vi "72 MP_Setting a servo.vi"() -> ()   [LabVIEW 2024]
uses:
  <userlib>/1. Examples/_Subs/OpenDiagram/Open_XControl.xctl
  <vilib>/Instr/_visa.llb/VISA Configure Serial Port (Instr).vi
panel:
  in  "OpenDiag":refnum<vi>(xcontrol)
  out "position read":u8=100
  in  "Position":u8(slide)=98 scale=0.0..180.0
  in  "MicroPython code":string="'''\nhttps://docs.micropython.org/en/latest/pyboard/tutorial/servo.html\n     \nconnections: \nGround (B) - GND \nPower  (R)   - 3V3 \nNC\nSignal -  pin X1\n'''\n\nimport pyb,utime,machine\n\nmachine.Pin('EN_3V3').on()\n\nusb = pyb.USB_VCP()\nservo1 = pyb.Servo(1)   # pix X1 \n\nwhile True:\n     utime.sleep_ms(10)\n     if usb.any():\n          reply = ord(usb.read())\n          #set the angle\n          servo1.angle(reply)\n          usb.send('%d \\n'%(reply))"
  in  "stop":bool
  out "Connected":bool
  in  "MicroPython Port":refnum<visa-resource-name>="ASRL96::INSTR"
  # "02 MicroPython Setting a Servo\nThis code takes will send a desired angle out to the device\n\nInstructions:\n1. Download the MicroPython Code into your device by saving it as main.py on your device\n2. restart your device\n3. Select the device port \n4. Hit Run - and watch the servo change position when you move the slider"
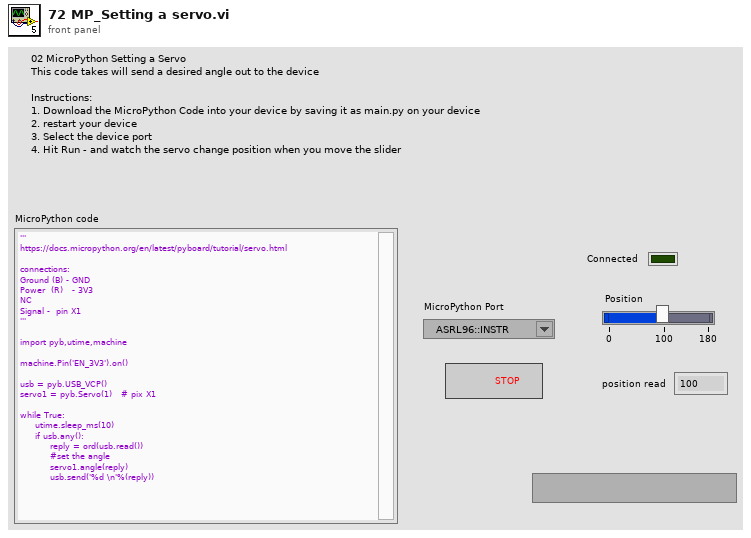
[diagram p1: front panel]
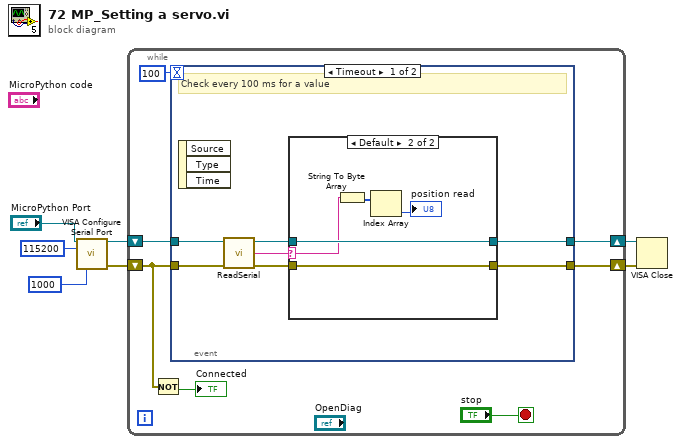
[diagram p0: block diagram]
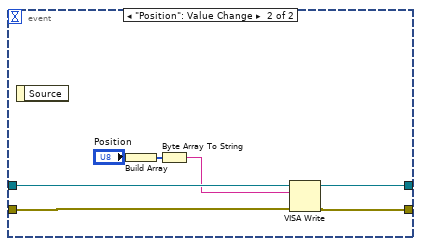
[diagram p3: hidden frame]
diagram:
  n1 = call-poly "VISA Configure Serial Port"("VISA resource name"="MicroPython Port", "timeout (10sec)"=u32 1000, "baud rate (9600)"=u32 115200) -> ("VISA resource name out"=w6:refnum<visa-resource-name>, "error out"=w5:errorcluster)  [unwired: 11 in]
  n2 = while {
    shift-right: [w12] -> w3
    shift-left: w6 -> [w14]
    shift-right: [w13] -> w4
    shift-left: w5 -> [w10]
    stop <- "stop" stop-if-true
    n3 = Not(x=w10) -> (.not. x?=→"Connected":bool)
    n4 = event shown="[0] Timeout" {
      selector: _ -> [_ _]
      dyn-events: _ -> [_ _]
      timeout: 100 -> [_ _]
      tunnel: w14 -> [w19 w35]
      tunnel: [w21 w33] -> w13
      tunnel: [w20 w32] -> w12
      tunnel: w10 -> [w18 w34]
      event Timeout {
        # "Check every 100 ms for a value"
        n5 = event-data() -> ()  [unwired: 1 in, 3 out]
        n6 = call <userlib>:"ReadSerial.vi"("error in (no error)"=w18, "VISA Refnum in"=w19) -> ("error out"=w17:errorcluster, "String"=w15:string, "VISA Refnum out"=w16:refnum<visa-resource-name>)  [unwired: 7 in]
        n7 = case shown="Default" w15 {
          selector: w15 -> [_ w24]
          tunnel: w16 -> [w23 w26]
          tunnel: w17 -> [w22 w25]
          tunnel: [w22 w25] -> w21
          tunnel: [w23 w26] -> w20
          frame "" {
          }
          frame Default {
            n8 = String To Byte Array(string=w24) -> (unsigned byte array=w28:u8[])
            n9 = Index Array(array=w28) -> (element=→"position read":u8)  [unwired: 1 in]
          }
        }
      }
      event "Position": Value Change {
        n10 = event-data() -> ()  [unwired: 1 in, 1 out]
        n11 = Build Array("Position") -> (w30:u8[])
        n12 = Byte Array To String(unsigned byte array=w30) -> (string=w29:string)
        n13 = VISA Write(VISA resource name=w35, write buffer=w29, error in (no error)=w34) -> (VISA resource name out=w32:refnum<visa-resource-name>, error out=w33:errorcluster)  [unwired: 1 out]
      }
    }
  }
  n14 = VISA Close(VISA resource name=w3, error in (no error)=w4) -> ()  [unwired: 1 out]
